vi "Calibration_Equation_VI.vi"(11 "Dynamic Data in":dynamicdata(waveform)) -> (3 "Dynamic Data out":dynamicdata(waveform))   [LabVIEW 2020]
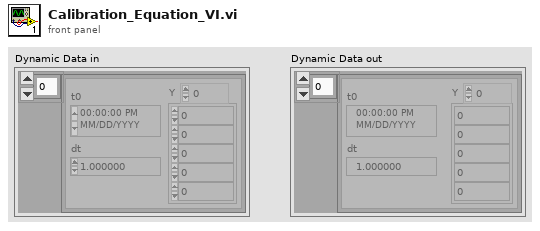
[diagram p1: front panel]
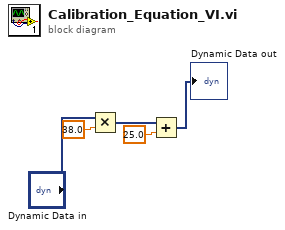
[diagram p0: block diagram]
diagram:
  n1 = Multiply(x="Dynamic Data in", y=38.0) -> (x*y=w3:dynamicdata)
  n2 = Add(x=w3, y=25.0) -> (x+y=→"Dynamic Data out":dynamicdata)
